vi "CODMn手动控制框.vi"(8 "Error in":errorcluster) -> ()   [LabVIEW 2016, in "斯坦道CODMn.lvlib"]
uses:
  <vilib>/Plasmionique/MB Master/MB Master.lvlib
panel:
  in  "高锰酸钾反滴定（10uL每滴）":bool
  in  "2#排":bool
  in  "2#进":bool
  in  "2#复位":bool
  in  "1#排":bool
  in  "1#进":bool
  in  "1#复位":bool
  in  "风扇":bool
  in  "排液":bool
  in  "搅拌":bool
  in  "加热":bool
  in  "硫酸":bool
  in  "加标回收样":bool
  in  "质控样":bool
  in  "标液":bool
  in  "纯水":bool
  in  "退出":bool
  in  "水样":bool
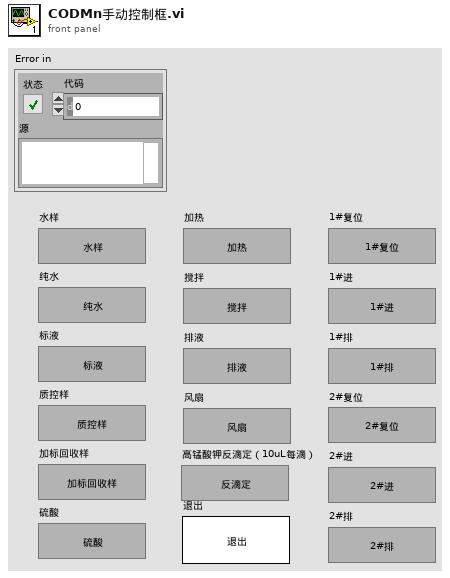
[diagram p1: front panel]
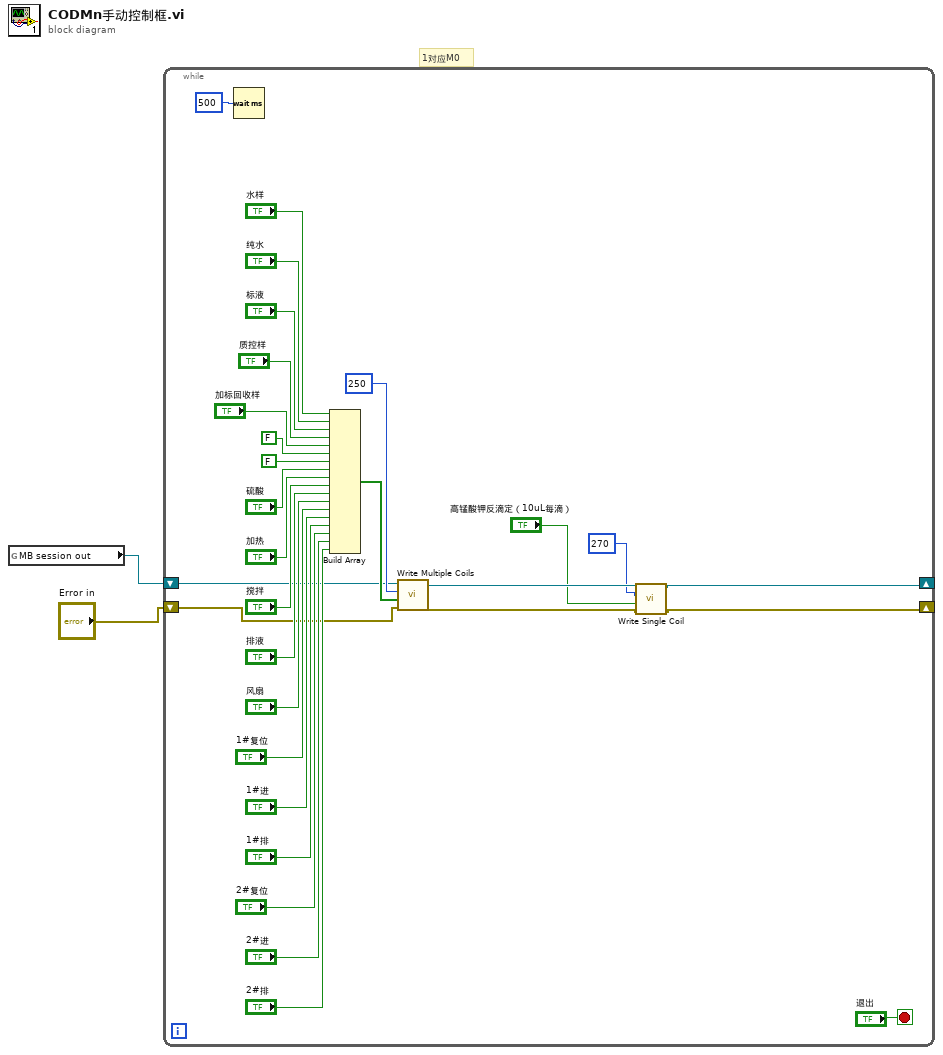
[diagram p0: block diagram]
diagram:
  # "1对应M0"
  n1 = global read "CODMn断电保存全局变量.vi" "MB session out"() -> (w1:refnum<class "MB_Master.lvclass">)
  n2 = while {
    shift-right: [w4] -> _
    shift-left: w1 -> [w10]
    shift-right: [w3] -> _
    shift-left: "Error in" -> [w9]
    stop <- "退出" stop-if-true
    n3 = Wait (ms)(milliseconds to wait=u32 500 ("等待时间（毫秒）")) -> ()  [unwired: 1 out]
    n4 = Build Array("水样", "纯水", "标液", "质控样", "加标回收样", FALSE ("元素"), FALSE ("元素"), "硫酸", "加热", "搅拌", "排液", "风扇", "1#复位", "1#进", "1#排", "2#复位", "2#进", "2#排") -> (w29:bool[])
    n5 = call <vilib>:"Write Multiple Coils.vi"("error in (no error)"=w9, "values"=w29, "starting address"=u16 250, "MB session in"=w10) -> ("error out"=w6:errorcluster, "MB session out"=w8:refnum<class "MB_Master.lvclass">)  [unwired: 6 in]
    n6 = call <vilib>:"Write Single Coil.vi"("error in (no error)"=w6, "value"="高锰酸钾反滴定（10uL每滴）", "address"=u16 270 ("starting address"), "MB session in"=w8) -> ("error out"=w3:errorcluster, "MB session out"=w4:refnum<class "MB_Master.lvclass">)  [unwired: 6 in]
  }
